vi "DMM Read Dual Display.vi"() -> ()   [LabVIEW 2011]
uses:
  <instrlib>/DMM4/DMM4.lvlib
panel:
  in  "Reset":bool
  out "Measure 2nd Value":string
  in  "Manual Range":dbl format="%#.9e"
  in  "Auto Range":bool=TRUE
  in  "2nd Function":u8(ring)=7 items=["DC Voltage", "AC Voltage", "DC Current", "AC Current", "2-Wire Resistance", "Frequency", "Period", "None"]
  in  "1st Function":u8(ring) items=["DC Voltage", "AC Voltage", "DC+AC Voltage", "DC Current", "AC Current", "DC+AC Current", "2-Wire Resistance", "Frequency", "Period", "Continuity", "Diode", "Temperature", "Capacitance"]
  out "error out":errorcluster
  out "Measure 1st Value":string
  in  "Stop":bool
  out "Boolean":bool
  in  "Detector Rate":u16(ring) items=["SLOW", "MID", "FAST"]
  in  "Manual Range":dbl format="%#.9e"
  in  "Auto Range":bool=TRUE
  out "ID Return String":string
  in  "Configure RS232 Baud Rate":u32(ring)=115200 items=["9600"=9600, "19200"=19200, "38400"=38400, "57600"=57600, "115200"=115200]
  in  "VISA resource name":refnum<visa-resource-name>
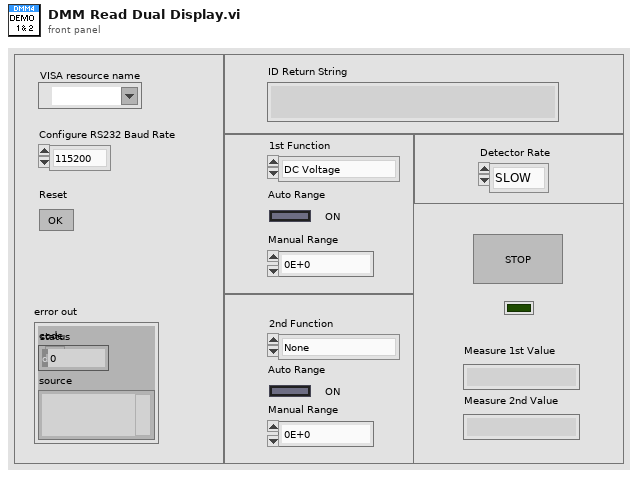
[diagram p1: front panel]
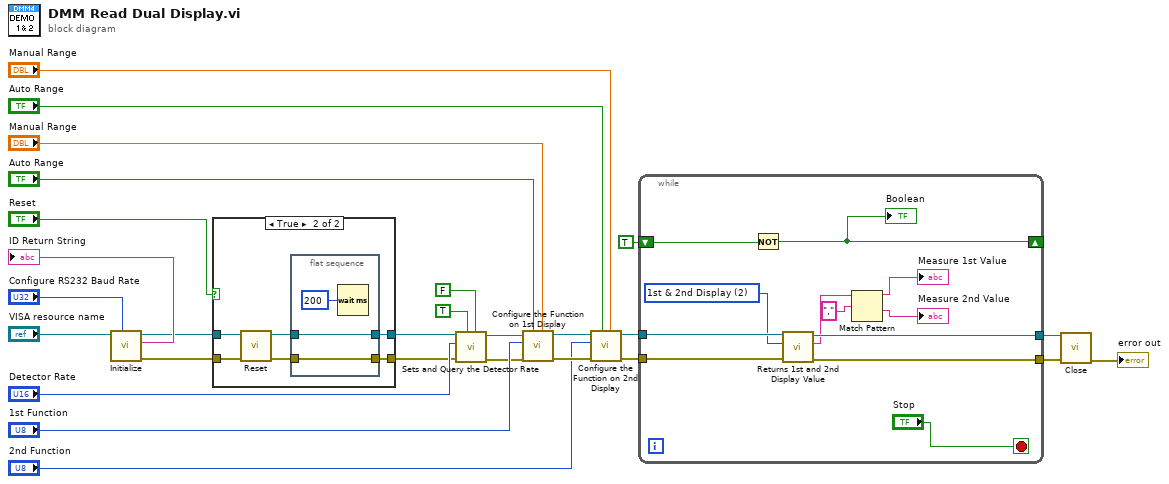
[diagram p0: block diagram]
diagram:
  n1 = call <instrlib>:"Initialize.vi"("Configure RS232 Baud Rate"="Configure RS232 Baud Rate", "VISA resource name"="VISA resource name") -> ("error out"=w18:errorcluster, "ID Return String"=→"ID Return String":string, "VISA resource name out"=w19:refnum<visa-resource-name>)  [unwired: 6 in, 1 out]
  n2 = case shown="True" "Reset" {
    tunnel: w19 -> [w29 w35]
    tunnel: w18 -> [w28 w34]
    tunnel: [w29 w32] -> w2
    tunnel: [w28 w30] -> w1
    frame False {
    }
    frame True {
      n3 = call <instrlib>:"Reset.vi"("error in (no error)"=w34, "VISA resource name"=w35) -> ("error out"=w31:errorcluster, "VISA resource name out"=w33:refnum<visa-resource-name>)  [unwired: 8 in]
      n4 = flat-sequence {
        tunnel: w33 -> [w37]
        tunnel: [w37] -> w32
        tunnel: w31 -> [w36]
        tunnel: [w36] -> w30
        frame #0 {
          n5 = Wait (ms)(milliseconds to wait=u32 200) -> ()  [unwired: 1 out]
        }
      }
    }
  }
  n6 = call <instrlib>:"Sets and Query the Detector Rate.vi"("Enable to Query"=FALSE, "Enable to Sets"=TRUE, "error in"=w1, "Detector Rate"="Detector Rate", "VISA resource name"=w2) -> ("error out"=w7:errorcluster, "VISA resource name out"=w8:refnum<visa-resource-name>)  [unwired: 4 in, 1 out]
  n7 = call <instrlib>:"Configure the Function on 1st Display .vi"("Manual Range"="Manual Range", "Enable Auto Range"="Auto Range", "error in"=w7, "Function"="1st Function", "VISA resource name"=w8) -> ("error out"=w15:errorcluster, "VISA resource name out"=w16:refnum<visa-resource-name>)  [unwired: 5 in]
  n8 = call <instrlib>:"Configure the Function on 2nd Display.vi"("Manual Range"="Manual Range", "Enable Auto Range"="Auto Range", "error in"=w15, "Function"="2nd Function", "VISA resource name"=w16) -> ("error out"=w9:errorcluster, "VISA resource name out"=w10:refnum<visa-resource-name>)  [unwired: 5 in]
  n9 = while {
    tunnel: w10 -> [w50]
    tunnel: w9 -> [w49]
    tunnel: [w46] -> w22
    tunnel: [w45] -> w21
    shift-right: [w43] -> _
    shift-left: TRUE -> [w44]
    stop <- "Stop" stop-if-true
    w48 = u16 2 items=["1st Display", "2nd Display", "1st & 2nd Display"] ("Sets to Display")
    n10 = Not(x=w44) -> (.not. x?=w43:bool)
    "Boolean" <- w43
    n11 = call <instrlib>:"Returns 1st and 2nd Display Value.vi"("error in"=w49, "Sets to Display"=w48, "VISA resource name"=w50) -> ("error out"=w45:errorcluster, "Return the Value"=w42:string, "VISA resource name out"=w46:refnum<visa-resource-name>)  [unwired: 6 in]
    n12 = Match Pattern(string=w42, regular expression=",") -> (before substring=→"Measure 1st Value":string, after substring=→"Measure 2nd Value":string)  [unwired: 1 in, 2 out]
  }
  n13 = call <instrlib>:"Close.vi"("error in (no error)"=w21, "VISA resource name"=w22) -> ("error out"=→"error out":errorcluster)  [unwired: 9 in]
